vi "wrap.TableNext.vi"(0 "class.GLue in":refnum<class "class.GLue.lvclass">, 11 "error in (no error)":errorcluster, 13 "Index":i32) -> (4 "class.GLue out":refnum<class "class.GLue.lvclass">, 8 "Return":i32, 15 "error out":errorcluster)   [LabVIEW 2014, in "GLue.lvlib" / "class.GLue.lvclass"]
uses:
  class.GLue.lvclass
  class.GLue.lvclass/class.GLue.ctl
  Resources/GLue.dll
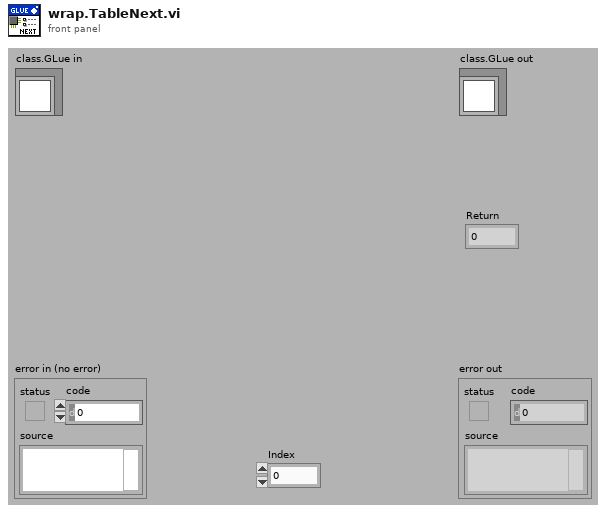
[diagram p1: front panel]
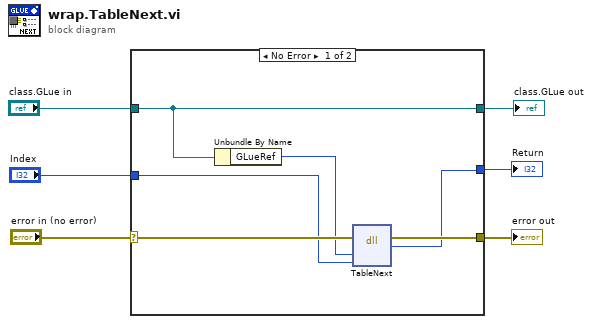
[diagram p0: block diagram]
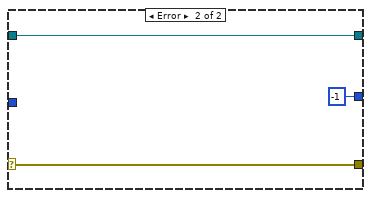
[diagram p2: hidden frame]
diagram:
  n1 = case shown="No Error" "error in (no error)" {
    selector: "error in (no error)" -> [w11 w15]
    tunnel: [w10 w15] -> w5
    tunnel: [w12 w14] -> w3
    tunnel: "class.GLue in" -> [w12 w14]
    tunnel: [w7 -1 ("Size")] -> w1
    tunnel: "Index" -> [w8 _]
    frame No Error {
      n2 = Unbundle By Name(w12) -> ("GLueRef"=w9:i64)
      n3 = dll-call lib="C:/Users/Antonie/Documents/work/glue/trunk/Resources/GLue.dll" fn="TableNext"(error in=w11, "MLua"=w9, "Index"=w8) -> (error out=w10:errorcluster, "Return"=w7:i32)  [unwired: 4 in, 1 out]
    }
    frame Error {
    }
  }
  "error out" <- w5
  "class.GLue out" <- w3
  "Return" <- w1
